vi "Minify JSON.vi"(10 "JSON String":string) -> (2 "Minified JSON":string)   [LabVIEW 2017, in "JSON.lvlib"]
uses:
  JSON.lvlib
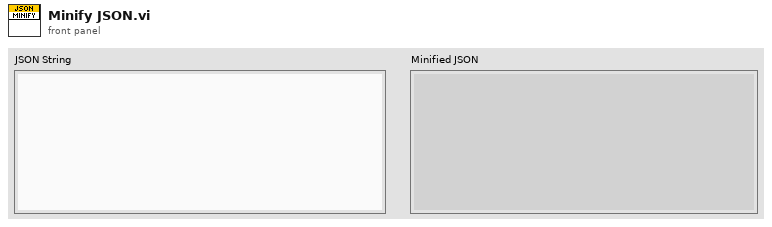
[diagram p1: front panel]
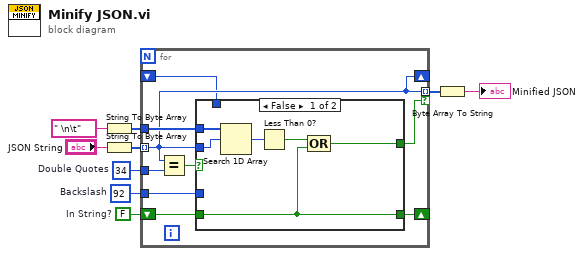
[diagram p0: block diagram]
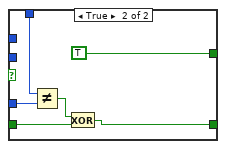
[diagram p2: hidden frame]
diagram:
  w3 = u8 92  # Backslash
  w5 = FALSE  # In String?
  w4 = u8 34  # Double Quotes
  n1 = String To Byte Array(string=" \n\t") -> (unsigned byte array=w6:u8[])
  n2 = String To Byte Array(string="JSON String") -> (unsigned byte array=w7:u8[])
  n3 = for {
    tunnel: w7 -> [w12] mode=indexing
    tunnel: w6 -> [w15]
    shift-right: [w13] -> _
    shift-left: w5 -> [w17]
    tunnel: w4 -> [w18]
    tunnel: [w12] -> w2 mode=indexing if=w14
    shift-right: [w12] -> _
    shift-left: _ -> [w11]
    tunnel: w3 -> [w10]
    n4 = Equal?(x=w12, y=w18) -> (x = y?=w16:bool)
    n5 = case shown="False" w16 {
      tunnel: w17 -> [w21 w27]
      tunnel: w15 -> [w24 _]
      tunnel: w12 -> [w23 _]
      tunnel: [w19 TRUE] -> w14
      tunnel: [w21 w26] -> w13
      tunnel: w11 -> [_ w28]
      tunnel: w10 -> [_ w29]
      frame False {
        n6 = Search 1D Array(1D array=w24, element=w23) -> (index of element=w22:i32)  [unwired: 1 in]
        n7 = Less Than 0?(x=w22) -> (x < 0?=w20:bool)
        n8 = Compound Arithmetic op=OR(w20, w21) -> (w19:bool)
      }
      frame True {
        n9 = Not Equal?(x=w28, y=w29) -> (x != y?=w25:bool)
        n10 = Exclusive Or(1:w27, 2:w25) -> (0:w26:bool)
      }
    }
  }
  n11 = Byte Array To String(unsigned byte array=w2) -> (string=→"Minified JSON":string)
